vi "Set Photon Counting Divisions.vi"(10 "divisions":i32, 11 "noOfDivisions":u32) -> (2 "divisions out":i32, 3 "function return":u32)   [LabVIEW 2018, in "AndorSDK.lvlib"]
doc: "EXPNETTYPE unsigned int WINAPI SetPhotonCountingDivisions(at_u32 noOfDivisions, at_32 * divisions);"
uses:
  AndorSDK.lvlib
  ATMCD32D.dll
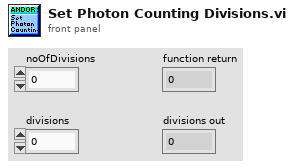
[diagram p1: front panel]
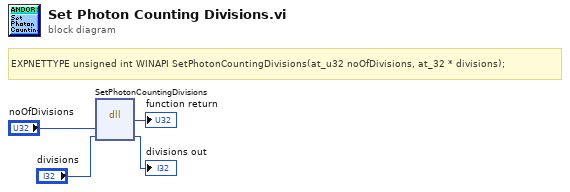
[diagram p0: block diagram]
diagram:
  # "EXPNETTYPE unsigned int WINAPI SetPhotonCountingDivisions(at_u32 noOfDivisions, at_32 * divisions);"
  n1 = dll-call lib="PTH2babs E\nPersönliches02 - Arbeit03-HiwijobsLabviewCodelibANDOR\tAndor SDK\nATMCD32D.*" fn="SetPhotonCountingDivisions"("noOfDivisions"="noOfDivisions", "divisions"="divisions") -> (→"function return":u32, "divisions"=→"divisions out":i32)  [unwired: 4 in, 2 out]
